vi "Create VIs.vi"(7 "Path":path, 9 "Property in":refnum<vi>, 10 "Template":refnum<vi>, 11 "prefix":string) -> (2 "Poly Info":T1(array[cluster]))   [LabVIEW 2015]
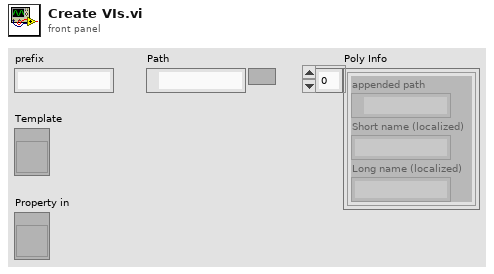
[diagram p1: front panel]
types:
  T1 = cluster{"appended path":path, "Short name (localized)":string, "Long name (localized)":string}[]
  T2 = typedef "ASPM_ArrayOfUniqueIDStringDatanameShortnameLongname.ctl" = T3[]
  T3 = typedef "ASPM_UniqueIDStringDatanameShortnameLongname.ctl" = cluster{"Unique ID string":string, "Data name":string, "Short name (localized)":string, "Long name (localized)":string}
  T4 = cluster{"appended path":path, "Short name (localized)":string, "Long name (localized)":string}
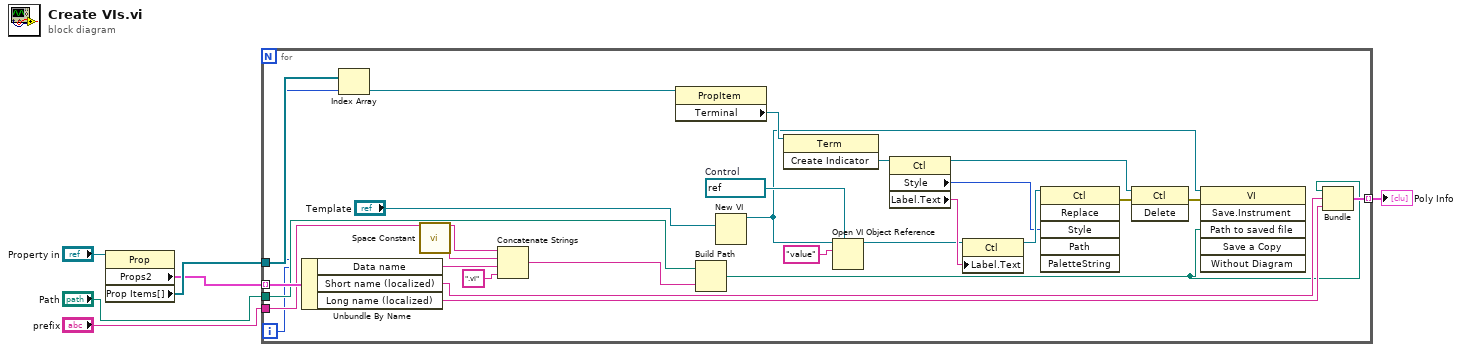
[diagram p0: block diagram]
diagram:
  n1 = property class="Prop"(reference="Property in") -> ("Props2"=w4:T2, "Prop Items[]"=w5:refnum<vi>[])  [unwired: 1 in, 2 out]
  n2 = for {
    tunnel: w5 -> [w24]
    tunnel: w4 -> [w23] mode=indexing
    tunnel: "Path" -> [w21]
    tunnel: "prefix" -> [w20]
    tunnel: [w13] -> w1 mode=indexing
    i -> [w9]
    w26 = refnum<vi> refnum  # Control
    n3 = Unbundle By Name(w23) -> ("Data name"=w18:string, "Short name (localized)"=w15:string, "Long name (localized)"=w14:string)
    n4 = Index Array(array=w24, index=w9) -> (element=w10:refnum<vi>)
    n5 = call <vilib>:"Space Constant.vi"() -> ("String"=w19:string)
    n6 = Concatenate Strings(w20, w19, w18, ".vi" ("string")) -> (w16:string)
    n7 = property class="PropItem"(reference=w10) -> ("Terminal"=w31:refnum<vi>)  [unwired: 1 in, 2 out]
    n8 = Build Path(base path=w21, name or relative path=w16) -> (appended path=w11:path)
    n9 = New VI(10:"Template") -> (3:w8:refnum<vi>)  [unwired: 6 in, 1 out]
    n10 = invoke class="Term" method="Create Indicator"(reference=w31) -> ("Create Indicator"=w7:refnum<vi>)  [unwired: 2 in, 2 out]
    n11 = Open VI Object Reference(7:w26, 10:"value" ("name/order"), 11:w8) -> (3:w28:refnum<vi>)  [unwired: 1 in, 1 out]
    n12 = property class="Ctl"(reference=w7) -> (reference out=w33:refnum<vi>, "Style"=w27:u32, "Label.Text"=w30:string)  [unwired: 1 in, 1 out]
    n13 = property class="Ctl"(reference=w28, "Label.Text"=w30) -> (reference out=w29:refnum<vi>)  [unwired: 1 in, 1 out]
    n14 = invoke class="Ctl" method="Replace"(reference=w29, "Style"=w27) -> (error out=w32:errorcluster)  [unwired: 4 in, 5 out]
    n15 = invoke class="Ctl" method="Delete"(reference=w33, error in=w32) -> (error out=w12:errorcluster)  [unwired: 1 in, 2 out]
    n16 = invoke class="VI" method="Save.Instrument"(reference=w8, error in=w12, "Path to saved file"=w11) -> ()  [unwired: 3 in, 6 out]
    n17 = Bundle("appended path"=w11, "Short name (localized)"=w15, "Long name (localized)"=w14) -> (w13:T4)  [unwired: 1 in]
  }
  "Poly Info" <- w1
